vi "Acceleromter_Gyroscope_9DOF(SPI_MPU9250).vi"() -> ()   [LabVIEW 2016]
uses:
  <vilib>/FPGAPlugInAG/myRIO-1900/niLvFpga_Open_myRIO-1900.vi
  <vilib>/rvi/interface/common/dynamic/niFpgaDynamicAddResources.vi
  <vilib>/Utility/error.llb/Error Cluster From Error Code.vi
  <vilib>/rvi/errors/niLvFpgaAdjustHostInterfaceError.vi
  <vilib>/rvi/interface/nirviOpenFPGA/nirviOpenFPGA.xnode
  FPGA Bitfiles/BalanceWheel_FPGATarget_MPUFPGA_wGUvAcQASr8.lvbitx
  MPU FPGA.vi
  <vilib>/rvi/interface/nirviReadWriteControl/nirviReadWriteControl.xnode
  <vilib>/rvi/interface/Simulation/niFpgaSimulationCallBeginRW.vi
  NiFpgaLv.dll
panel:
  in  "stop data collection":bool
  in  "Stop offset":bool
  in  "?":bool
  in  "?":bool
  out "Offset locked":bool
  in  "Accelerometer\n range (g)":enum16{"16", "8", "4", "2"}(ring)
  in  "Gyroscope\n range (deg/s)":enum16{"2000", "1000", "500", "250"}(ring)
  out "Acceleration (g)":cluster{dbl, dbl, dbl}(graph)
  out "Gyroscope (deg/s)":cluster{dbl, dbl, dbl}(graph)
  out "Compass":cluster{dbl, dbl, dbl}(graph)
  out "XAOffset":dbl
  out "YAOffset":dbl
  out "ZAOffset":dbl
  out "XGOffset":dbl
  out "YGOffset":dbl
  out "ZGOffset":dbl
  out "Acceleration (g)":cluster{dbl, dbl, dbl}(graph)
  out "Gyroscope\n(deg/s)":cluster{dbl, dbl, dbl}(graph)
  out "Compass (deg)":cluster{dbl, dbl, dbl}(graph)
  out "ZAOff1":dbl
  out "YAOff1":dbl
  out "XAOff1":dbl
  out "Iterations took\nto achieve offset":i32
  out "XGOff":dbl
  out "YGOff":dbl
  out "ZGOff":dbl
  out "output array":u16[](array[numeric])
  out "Array":u16[](array[numeric])=[5119, 5120, 5630, 5823, 5888, 6198, 6419, 6658, 6912, 7176, 7430, 7680, 7936, 8960, 14337, 14849, 27393, 30464, 30720, 31232, 31488, 32000, 32256, 27168, 26371, 6419, 6658, 14337, 14849, 9280, 9612, 9730, 10120, 10252, 10506, 10881, 25601, 27648]
  # "Range"
  # "Offset"
  # "Readings after offset achieved"
  # "Readings at offset"
  # "select the sensor range below, before you hit start"
  # "Turning off will increase \nthe speed of RT(real time processor/MyRIO)"
  # "X- White\nY- Red\nZ- Green"
  # "We are not offsetting compass"
  # "offset bits\nsent to the register (decimal)"
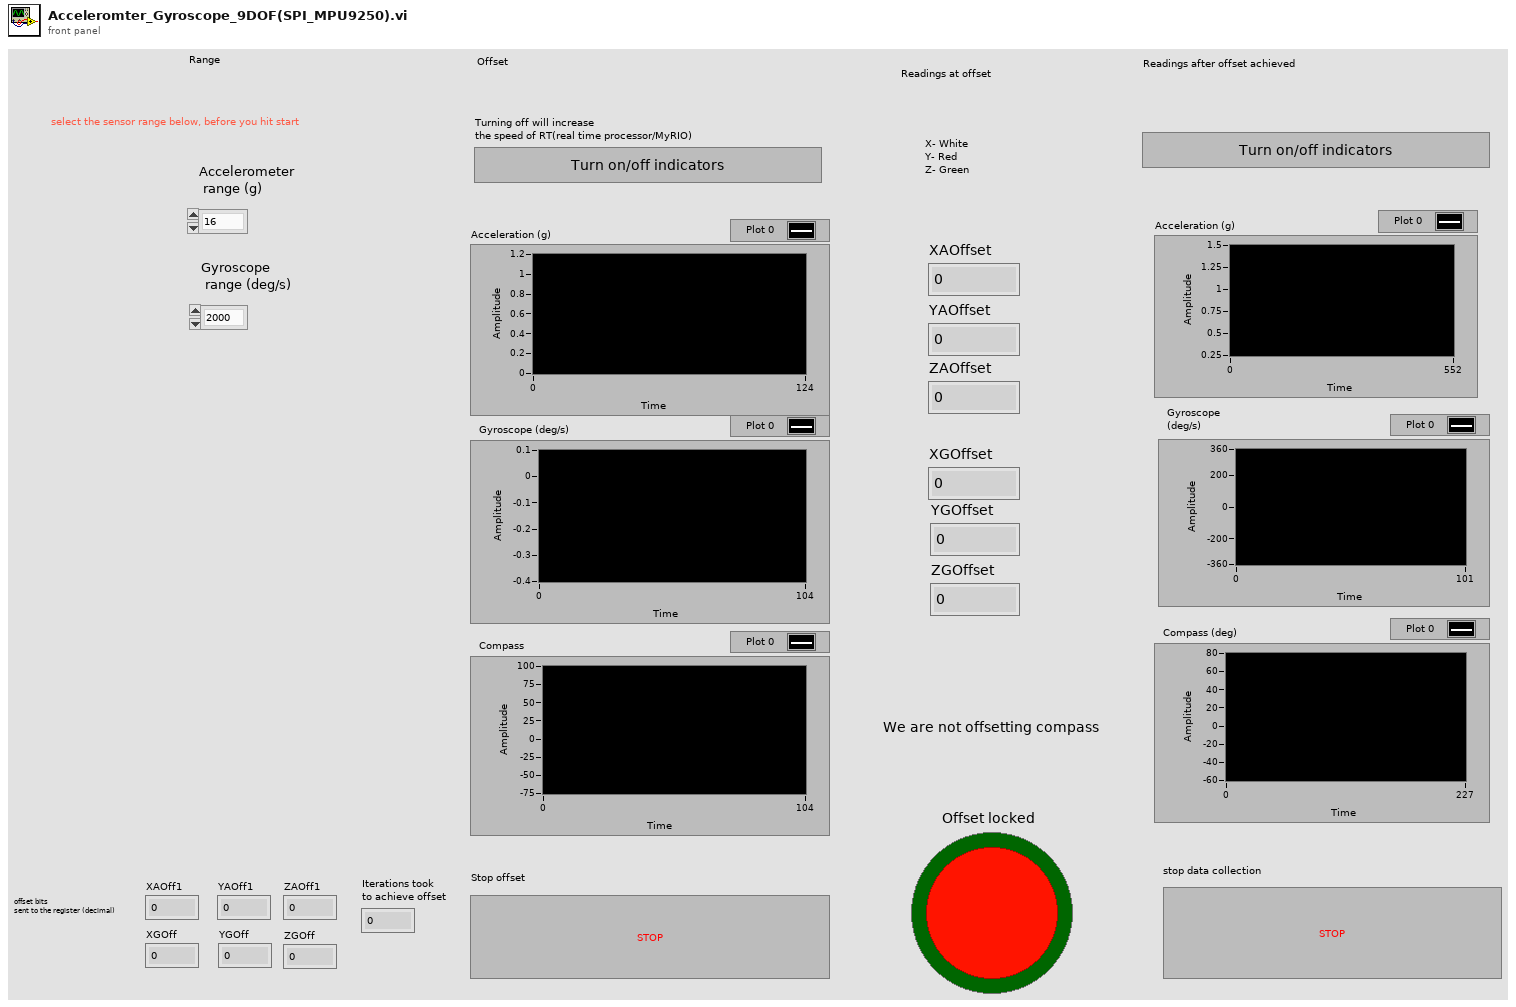
[diagram p1: front panel]
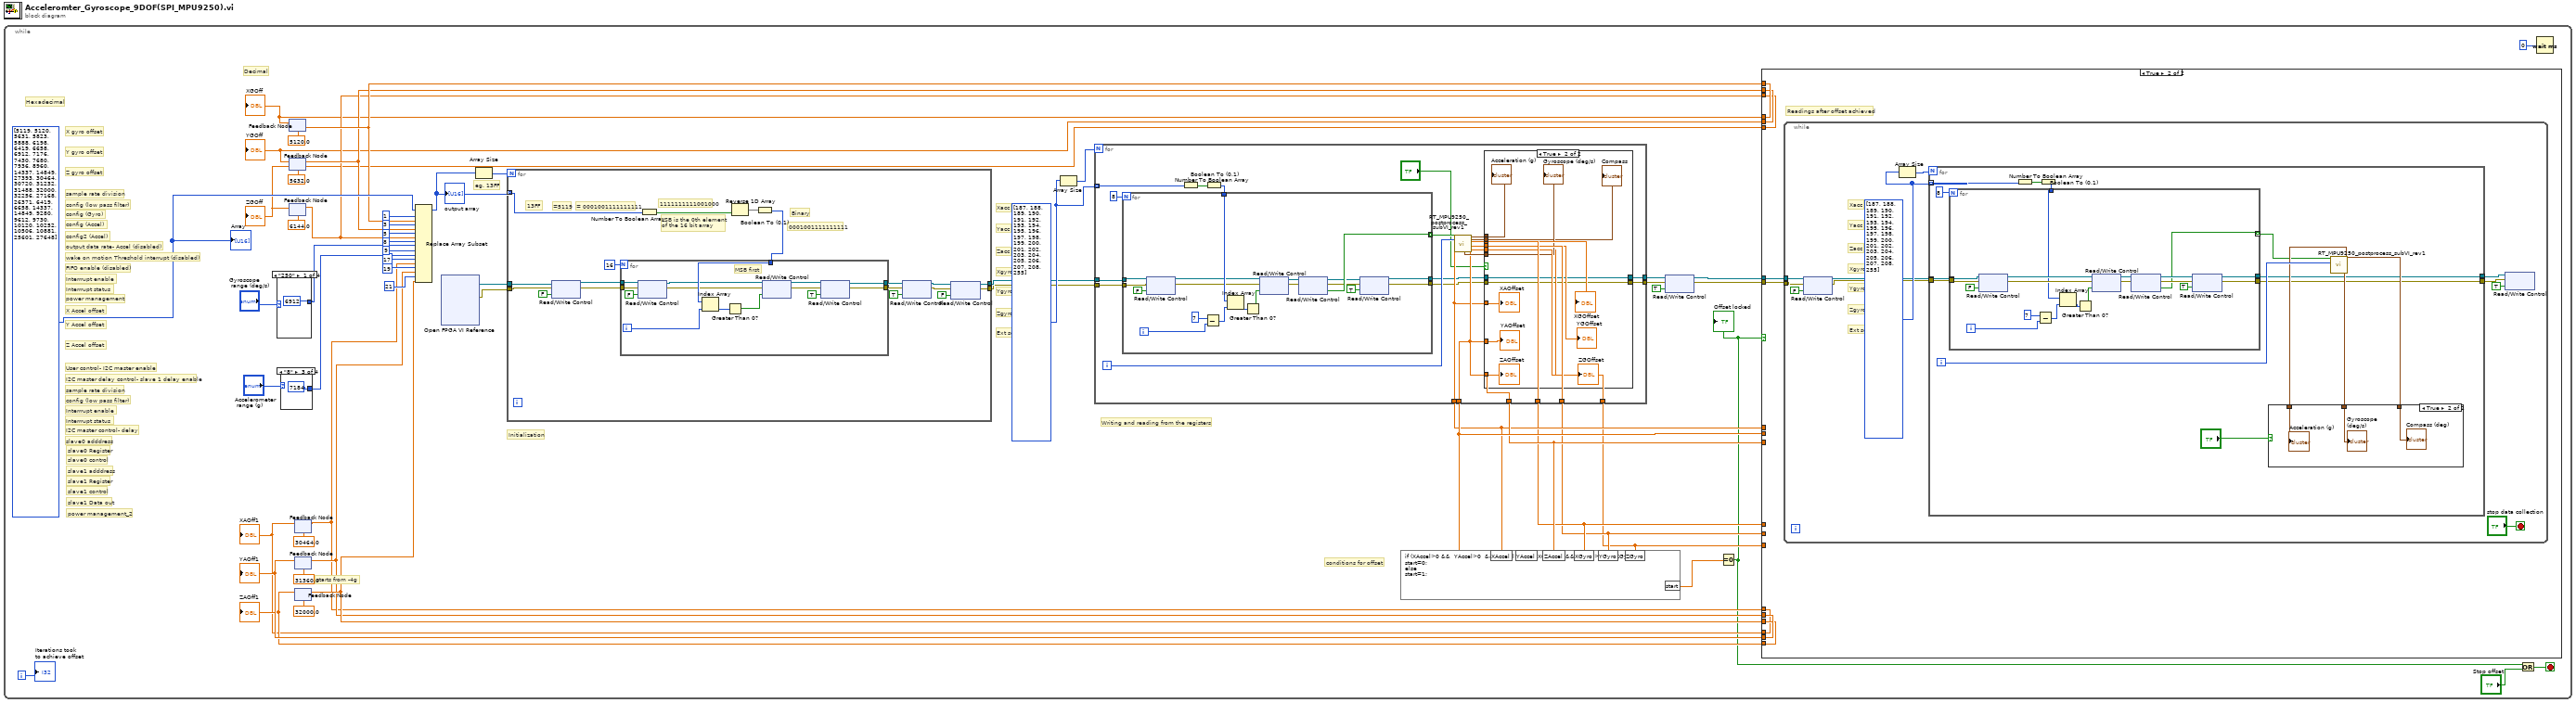
[diagram p0: block diagram]
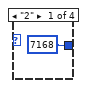
[diagram p2: hidden frame]
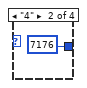
[diagram p3: hidden frame]
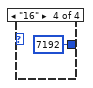
[diagram p4: hidden frame]
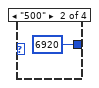
[diagram p5: hidden frame]
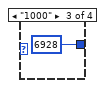
[diagram p6: hidden frame]
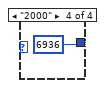
[diagram p7: hidden frame]
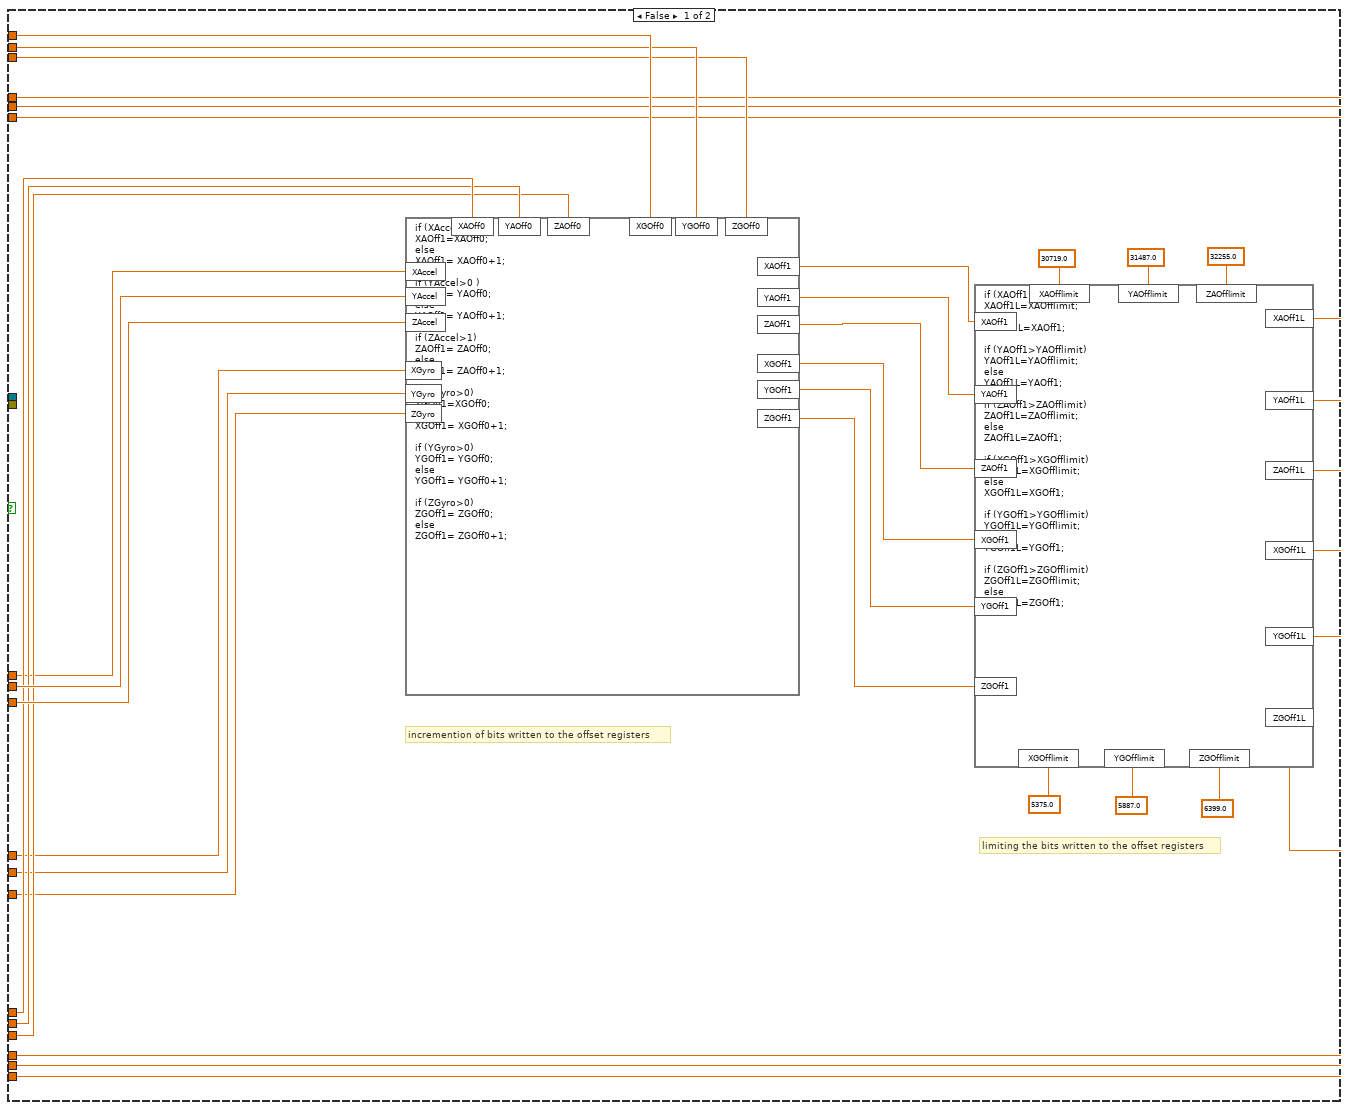
[diagram p8: hidden frame]
diagram:
  n1 = while {
    i -> [w43]
    stop <- w8 stop-if-true
    w25 = u16[] [187, 188, 189, 190, 191, 192, 193, 194, 195, 196, 197, 198, 199, 200, 201, 202, 203, 204, 205, 206, 207, 208, 255] ("Frames to Write")
    w38 = u16[] [5119, 5120, 5631, 5823, 5888, 6198, 6419, 6658, 6912, 7176, 7430, 7680, 7936, 8960, 14337, 14849, 27393, 30464, 30720, 31232, 31488, 32000, 32256, 27168, 26371, 6419, 6658, 14337, 14849, 9280, 9612, 9730, 10120, 10252, 10506, 10881, 25601, 27648]
    # "Decimal"
    # "Hexadecimal"
    # "conditions for offset"
    # "Writing and reading from the registers"
    # "Initialization"
    # "starts from -4g"
    # "7"
    # "6"
    # "5"
    # "4"
    # "3"
    # "2"
    # "1"
    # "Ext sens 0"
    # "Zgyro"
    # "Ygyro"
    # "Xgyro"
    # "Zacc"
    # "Yacc"
    # "Xacc"
    # "power management_2"
    # "slave1 Data out"
    # "slave1 control"
    # "slave1 Register"
    # "slave1 adddress"
    # "slave0 control"
    # "slave0 Register"
    # "slave0 adddress"
    # "I2C master control- delay"
    # "Interrrupt status"
    # "Interrrupt enable"
    # "config (low pass filter)"
    # "sample rate division"
    # "I2C master delay control- slave 1 delay enable"
    # "User control- I2C master enable"
    # "Z Accel offset"
    # "Y Accel offset"
    # "X Accel offset"
    # "power management"
    # "Interrrupt status"
    # "Interrrupt enable"
    # "FIFO enable (disabled)"
    # "wake on motion Threshold interrupt (disabled)"
    # "output data rate- Accel (disabled)"
    # "config2 (Accel)"
    # "config (Accel)"
    # "config (Gyro)"
    # "config (low pass filter)"
    # "sample rate division"
    # "Z gyro offset"
    # "Z gyro offset"
    # "Y gyro offset"
    # "X gyro offset"
    # "eg. 13FF"
    n2 = case shown="\"250\"" "Gyroscope\n range (deg/s)" {
      tunnel: [6912 6920 6928 6936] -> w23
      frame "250" {
      }
      frame "500" {
      }
      frame "1000" {
      }
      frame "2000" {
      }
    }
    n3 = case shown="\"8\"" "Accelerometer\n range (g)" {
      tunnel: [7168 7176 7184 7192] -> w13
      frame "2" {
      }
      frame "4" {
      }
      frame "8" {
      }
      frame "16" {
      }
    }
    n4 = feedback #1(5120.0 ("XAOff1")) -> (w31:dbl)
    n5 = feedback #2(5632.0 ("XAOff1")) -> (w30:dbl)
    n6 = feedback #3(6144.0 ("XAOff1")) -> (w29:dbl)
    n7 = feedback #4(30464.0 ("XAOff1")) -> (w17:dbl)
    n8 = feedback #5(31360.0 ("XAOff1")) -> (w19:dbl)
    n9 = feedback #6(32000.0 ("XAOff1")) -> (w21:dbl)
    n10 = Replace Array Subset(array=w38, new element #1=w31, index #1=1 ("index"), new element #2=w30, index #2=3 ("index"), new element #3=w29, index #3=5 ("index"), new element #4=w23, index #4=8 ("index"), new element #5=w13, index #5=9 ("index"), new element #6=w17, index #6=17 ("index"), new element #7=w19, index #7=19 ("index"), new element #8=w21, index #8=21 ("index")) -> (w39:u16[])
    "output array" <- w39
    n11 = xnode "Open FPGA VI Reference"() -> ("FPGA VI Reference Out"=w1:refnum<k20>, "error out"=w2:errorcluster)  [unwired: 2 in]
    n12 = Array Size(array=w39) -> (size(s)=w56:i32)
    n13 = for {
      N: w56 -> [_]
      tunnel: w39 -> [w221] mode=indexing
      tunnel: w1 -> [w216]
      tunnel: w2 -> [w215]
      tunnel: [w205] -> w12
      tunnel: [w204] -> w11
      # "Binary"
      # "13FF"
      # "0001001111111111"
      # "1111111111001000"
      # "= 0001001111111111"
      # "LSB is the 0th element\nof the 16 bit array"
      # "=5119"
      n14 = xnode "Read/Write Control"("FPGA VI Reference In"=w216, "error in"=w215, "CS"=FALSE) -> ("FPGA VI Reference Out"=w214:refnum<k20>, "error out"=w213:errorcluster)
      n15 = Number To Boolean Array(number=w221) -> (Boolean array=w219:bool[])
      n16 = Reverse 1D Array(array=w219) -> (reversed array=w218:bool[])
      n17 = Boolean To (0,1)(Boolean=w218) -> (0, 1=w220:i16[])
      n18 = for {
        N: 16 -> [_]
        tunnel: w220 -> [w234]
        tunnel: w214 -> [w232]
        tunnel: w213 -> [w231]
        tunnel: [w223] -> w210
        tunnel: [w222] -> w209
        i -> [w235]
        # "MSB first"
        n19 = xnode "Read/Write Control"("FPGA VI Reference In"=w232, "error in"=w231, "SCL"=FALSE) -> ("FPGA VI Reference Out"=w228:refnum<k20>, "error out"=w227:errorcluster)
        n20 = Index Array(array=w234, index=w235) -> (element=w233:i16)
        n21 = Greater Than 0?(x=w233) -> (x > 0?=w229:bool)
        n22 = xnode "Read/Write Control"("FPGA VI Reference In"=w228, "error in"=w227, "MOSI"=w229) -> ("FPGA VI Reference Out"=w225:refnum<k20>, "error out"=w224:errorcluster)
        n23 = xnode "Read/Write Control"("FPGA VI Reference In"=w225, "error in"=w224, "SCL"=TRUE) -> ("FPGA VI Reference Out"=w223:refnum<k20>, "error out"=w222:errorcluster)
      }
      n24 = xnode "Read/Write Control"("FPGA VI Reference In"=w210, "error in"=w209, "CS"=TRUE) -> ("FPGA VI Reference Out"=w207:refnum<k20>, "error out"=w206:errorcluster)
      n25 = xnode "Read/Write Control"("FPGA VI Reference In"=w207, "error in"=w206, "CS"=FALSE) -> ("FPGA VI Reference Out"=w205:refnum<k20>, "error out"=w204:errorcluster)
    }
    n26 = Array Size(array=w25) -> (size(s)=w54:i32)
    n27 = for {
      N: w54 -> [_]
      tunnel: w12 -> [w167]
      tunnel: w11 -> [w166]
      tunnel: w25 -> [w169] mode=indexing
      tunnel: [w159] -> w52
      tunnel: [w158] -> w51
      tunnel: [w157] -> w44
      tunnel: [w160] -> w32
      tunnel: [w161] -> w33
      tunnel: [w163] -> w34
      tunnel: [w151] -> w4
      tunnel: [w150] -> w3
      i -> [w165]
      n28 = Number To Boolean Array(number=w169) -> (Boolean array=w171:bool[])
      n29 = Boolean To (0,1)(Boolean=w171) -> (0, 1=w168:i16[])
      n30 = for {
        N: 8 -> [_]
        tunnel: [w190] -> w164 mode=indexing
        tunnel: w168 -> [w200]
        tunnel: w167 -> [w197]
        tunnel: w166 -> [w196]
        tunnel: [w188] -> w153
        tunnel: [w187] -> w152
        i -> [w203]
        n31 = xnode "Read/Write Control"("FPGA VI Reference In"=w197, "error in"=w196, "SCL"=FALSE) -> ("FPGA VI Reference Out"=w194:refnum<k20>, "error out"=w193:errorcluster)
        n32 = Subtract(x=7, y=w203) -> (x-y=w201:i32)
        n33 = Index Array(array=w200, index=w201) -> (element=w199:i16)
        n34 = Greater Than 0?(x=w199) -> (x > 0?=w195:bool)
        n35 = xnode "Read/Write Control"("FPGA VI Reference In"=w194, "error in"=w193, "MOSI"=w195) -> ("FPGA VI Reference Out"=w192:refnum<k20>, "error out"=w191:errorcluster)
        n36 = xnode "Read/Write Control"("FPGA VI Reference In"=w192, "error in"=w191) -> ("FPGA VI Reference Out"=w186:refnum<k20>, "error out"=w185:errorcluster, "MISO"=w190:bool)
        n37 = xnode "Read/Write Control"("FPGA VI Reference In"=w186, "error in"=w185, "SCL"=TRUE) -> ("FPGA VI Reference Out"=w188:refnum<k20>, "error out"=w187:errorcluster)
      }
      n38 = call "RT_MPU9250_postprocess_subVI_rev1.vi"("readings in bits"=w164, "number of samples"=w165) -> ("Zgyro"=w160:dbl, "Ygyro"=w161:dbl, "XAccel"=w157:dbl, "Gyroscope (deg/s)"=w162:cluster{dbl, dbl, dbl}, "Xgyro"=w163:dbl, "Acceleration (g)"=w156:cluster{dbl, dbl, dbl}, "Compass"=w155:cluster{dbl, dbl, dbl}, "YAccel"=w159:dbl, "ZAccel"=w158:dbl)  [unwired: 5 in, 4 out]
      n39 = case shown="True" "?" {
        tunnel: w163 -> [_ w184]
        tunnel: w162 -> [_ w183]
        tunnel: w161 -> [_ w182]
        tunnel: w160 -> [_ w181]
        tunnel: w159 -> [_ w180]
        tunnel: w158 -> [_ w179]
        tunnel: w157 -> [_ w178]
        tunnel: w156 -> [_ w177]
        tunnel: w155 -> [_ w176]
        tunnel: w153 -> [w173 w175]
        tunnel: w152 -> [w172 w174]
        tunnel: [w173 w175] -> w151
        tunnel: [w172 w174] -> w150
        frame False {
        }
        frame True {
          "Acceleration (g)" <- w177
          "Gyroscope (deg/s)" <- w183
          "Compass" <- w176
          "XAOffset" <- w178
          "YAOffset" <- w180
          "ZAOffset" <- w179
          "XGOffset" <- w184
          "YGOffset" <- w182
          "ZGOffset" <- w181
        }
      }
    }
    n40 = formula code="if (XAccel>0 &&  YAccel>0  && ZAccel>1 &&  XGyro>0 && YGyro>0 && ZGyro>0)\nstart=0; \nelse\nstart=1;"("XAccel"=w44, "YAccel"=w52, "ZAccel"=w51, "XGyro"=w34, "YGyro"=w33, "ZGyro"=w32) -> ("start"=w53:dbl)
    n41 = xnode "Read/Write Control"("FPGA VI Reference In"=w4, "error in"=w3, "CS"=TRUE) -> ("FPGA VI Reference Out"=w6:refnum<k20>, "error out"=w5:errorcluster)
    n42 = Equal To 0?(x=w53) -> (x = 0?=w10:bool)
    "Offset locked" <- w10
    n43 = case shown="True" w10 {
      tunnel: w6 -> [_ w102]
      tunnel: w5 -> [_ w101]
      tunnel: w52 -> [w94 _]
      tunnel: w51 -> [w93 _]
      tunnel: [w73 w100] -> w49
      tunnel: [w71 w99] -> w47
      tunnel: w17 -> [w92 w98]
      tunnel: w19 -> [w91 w100]
      tunnel: w21 -> [w90 w99]
      tunnel: [w74 w98] -> w45
      tunnel: w44 -> [w89 _]
      tunnel: w34 -> [w88 _]
      tunnel: w33 -> [w87 _]
      tunnel: w32 -> [w86 _]
      tunnel: [w78 w97] -> w28
      tunnel: [w77 w96] -> w26
      tunnel: [w75 w95] -> w27
      tunnel: w31 -> [w85 w97]
      tunnel: w30 -> [w84 w96]
      tunnel: w29 -> [w83 w95]
      frame False {
        # "limiting the bits written to the offset registers"
        # "incremention of bits written to the offset registers"
        n44 = formula code="if (XAccel>0)\nXAOff1=XAOff0;\nelse\nXAOff1= XAOff0+1;\n\nif (YAccel>0 )\nYAOff1= YAOff0;\nelse\nYAOff1= YAOff0+1;\n\nif (ZAccel>1)\nZAOff1= ZAOff0;\nelse\nZAOff1= ZAOff0+1;\n\nif (XGyro>0)\nXGOff1=XGOff0;\nelse\nXGOff1= XGOff0+1;\n\nif (YGyro>0)\nYGOff1= YGOff0;\nelse\nYGOff1= YGOff0+1;\n\nif (ZGyro>0)\nZGOff1= ZGOff0;\nelse\nZGOff1= ZGOff0+1;"("XAOff0"=w92, "XAccel"=w89, "YAccel"=w94, "ZAccel"=w93, "YAOff0"=w91, "ZAOff0"=w90, "XGyro"=w88, "YGyro"=w87, "ZGyro"=w86, "XGOff0"=w85, "YGOff0"=w84, "ZGOff0"=w83) -> ("YAOff1"=w81:dbl, "ZAOff1"=w72:dbl, "XAOff1"=w82:dbl, "XGOff1"=w80:dbl, "YGOff1"=w79:dbl, "ZGOff1"=w76:dbl)
        n45 = formula code="if (XAOff1>XAOfflimit)\nXAOff1L=XAOfflimit;\nelse\n XAOff1L=XAOff1;\n\nif (YAOff1>YAOfflimit)\nYAOff1L=YAOfflimit;\nelse \nYAOff1L=YAOff1;\n\nif (ZAOff1>ZAOfflimit)\nZAOff1L=ZAOfflimit;\nelse \nZAOff1L=ZAOff1;\n\nif (XGOff1>XGOfflimit)\nXGOff1L=XGOfflimit;\nelse \nXGOff1L=XGOff1;\n\nif (YGOff1>YGOfflimit)\nYGOff1L=YGOfflimit;\nelse \nYGOff1L=YGOff1;\n\nif (ZGOff1>ZGOfflimit)\nZGOff1L=ZGOfflimit;\nelse \nZGOff1L=ZGOff1;"("XGOff1"=w80, "YGOff1"=w79, "ZGOff1"=w76, "XAOff1"=w82, "YAOff1"=w81, "ZAOff1"=w72, "XAOfflimit"=30719.0 ("input variable"), "YAOfflimit"=31487.0 ("input variable"), "ZAOfflimit"=32255.0 ("input variable"), "XGOfflimit"=5375.0 ("input variable"), "YGOfflimit"=5887.0 ("input variable"), "ZGOfflimit"=6399.0 ("input variable")) -> ("XAOff1L"=w74:dbl, "YAOff1L"=w73:dbl, "ZAOff1L"=w71:dbl, "XGOff1L"=w78:dbl, "YGOff1L"=w77:dbl, "ZGOff1L"=w75:dbl)
      }
      frame True {
        # "Readings after offset achieved"
        n46 = while {
          tunnel: w102 -> [w109]
          tunnel: w101 -> [w108]
          stop <- "stop data collection" stop-if-true
          w112 = u16[] [187, 188, 189, 190, 191, 192, 193, 194, 195, 196, 197, 198, 199, 200, 201, 202, 203, 204, 205, 206, 207, 208, 255] ("Frames to Write")
          # "7"
          # "6"
          # "5"
          # "4"
          # "3"
          # "2"
          # "1"
          # "Ext sens 0"
          # "Zgyro"
          # "Ygyro"
          # "Xgyro"
          # "Zacc"
          # "Yacc"
          # "Xacc"
          n47 = xnode "Read/Write Control"("FPGA VI Reference In"=w109, "error in"=w108, "CS"=FALSE) -> ("FPGA VI Reference Out"=w107:refnum<k20>, "error out"=w106:errorcluster)
          n48 = Array Size(array=w112) -> (size(s)=w113:i32)
          n49 = for {
            N: w113 -> [_]
            tunnel: w112 -> [w125] mode=indexing
            tunnel: w107 -> [w117]
            tunnel: w106 -> [w116]
            tunnel: [w115] -> w104
            tunnel: [w114] -> w103
            i -> [w123]
            n50 = Number To Boolean Array(number=w125) -> (Boolean array=w127:bool[])
            n51 = Boolean To (0,1)(Boolean=w127) -> (0, 1=w124:i16[])
            n52 = for {
              N: 8 -> [_]
              tunnel: [w133] -> w119 mode=indexing
              tunnel: w124 -> [w134]
              tunnel: w117 -> [w137]
              tunnel: w116 -> [w136]
              tunnel: [w132] -> w115
              tunnel: [w131] -> w114
              i -> [w135]
              n53 = xnode "Read/Write Control"("FPGA VI Reference In"=w137, "error in"=w136, "SCL"=FALSE) -> ("FPGA VI Reference Out"=w144:refnum<k20>, "error out"=w143:errorcluster)
              n54 = Subtract(x=7, y=w135) -> (x-y=w148:i32)
              n55 = Index Array(array=w134, index=w148) -> (element=w147:i16)
              n56 = Greater Than 0?(x=w147) -> (x > 0?=w145:bool)
              n57 = xnode "Read/Write Control"("FPGA VI Reference In"=w144, "error in"=w143, "MOSI"=w145) -> ("FPGA VI Reference Out"=w142:refnum<k20>, "error out"=w141:errorcluster)
              n58 = xnode "Read/Write Control"("FPGA VI Reference In"=w142, "error in"=w141) -> ("FPGA VI Reference Out"=w139:refnum<k20>, "error out"=w138:errorcluster, "MISO"=w133:bool)
              n59 = xnode "Read/Write Control"("FPGA VI Reference In"=w139, "error in"=w138, "SCL"=TRUE) -> ("FPGA VI Reference Out"=w132:refnum<k20>, "error out"=w131:errorcluster)
            }
            n60 = call "RT_MPU9250_postprocess_subVI_rev1.vi"("readings in bits"=w119, "number of samples"=w123) -> ("Gyroscope (deg/s)"=w120:cluster{dbl, dbl, dbl}, "Acceleration (g)"=w121:cluster{dbl, dbl, dbl}, "Compass"=w122:cluster{dbl, dbl, dbl})  [unwired: 5 in, 10 out]
            n61 = case shown="True" "?" {
              tunnel: w122 -> [_ w130]
              tunnel: w121 -> [_ w129]
              tunnel: w120 -> [_ w128]
              frame False {
              }
              frame True {
                "Acceleration (g)" <- w129
                "Gyroscope\n(deg/s)" <- w128
                "Compass (deg)" <- w130
              }
            }
          }
          n62 = xnode "Read/Write Control"("FPGA VI Reference In"=w104, "error in"=w103, "CS"=TRUE) -> ()  [unwired: 2 out]
        }
      }
    }
    "ZAOff1" <- w47
    "YAOff1" <- w49
    "XAOff1" <- w45
    "XGOff" <- w28
    "YGOff" <- w26
    "ZGOff" <- w27
    n63 = feedback-in #1(w28) -> ()
    n64 = feedback-in #2(w26) -> ()
    n65 = feedback-in #3(w27) -> ()
    n66 = feedback-in #4(w45) -> ()
    n67 = feedback-in #5(w49) -> ()
    n68 = feedback-in #6(w47) -> ()
    n69 = Or(x=w10, y="Stop offset") -> (x .or. y?=w8:bool)
    n70 = Wait (ms)(milliseconds to wait=u32 0) -> ()  [unwired: 1 out]
    "Iterations took\nto achieve offset" <- w43
    "Array" <- w38
  }
